vi "1820_LPF_ON_duration.vi"(10 "Lambda":bool, 11 "LPF ON":timestamp) -> (3 "LPF on (min)":dbl)   [LabVIEW 2016]
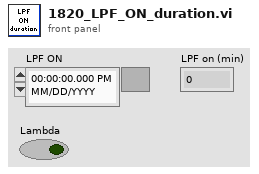
[diagram p1: front panel]
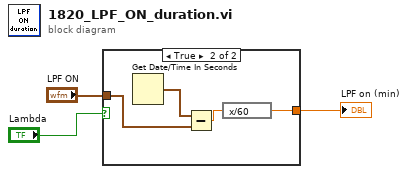
[diagram p0: block diagram]
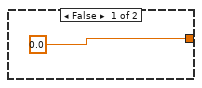
[diagram p2: hidden frame]
diagram:
  n1 = case shown="True" "Lambda" {
    tunnel: "LPF ON" -> [_ w5]
    tunnel: [0.0 ("LPF on (s)") w7] -> w3
    frame False {
    }
    frame True {
      n2 = Get Date/Time In Seconds() -> (seconds since 1Jan1904=w6:timestamp)
      n3 = Subtract(x=w6, y=w5) -> (x-y=w8:dbl)
      n4 = expression code="x/60"(w8) -> (w7:dbl)
    }
  }
  "LPF on (min)" <- w3
